vi "STP Protocol_Post_VI_Init.vi"(0 "object in":refnum<class "STP Protocol.lvclass">, 5 "Init Data":T1={"TxID"=0, "RxID"=0, "CMD"=0, "RQ Data"=[], "+veResponseCode"=160, "ResponseTimeout (S)"=0.1} {"ResponseTimeout (S)" format="%#_13g"; "+veResponseCode" format="%x"; "CMD" items=["TSW_VERSION(130)"=130, "WAIT_EVENT(132)"=132, "SEQUENCER(133)"=133, "TSW_RESET(150)"=150, "CONFIG_ECU(151)"=151, "TEST_CORE (152)"=152, "TEST_WATCHDOG (153)"=153, "TEST_MONITORING (154)"=154, "READ_MEMORY (162)"=162, "WRITE_ERASE_MEMORY (164)"=164, "COMM_EXTERNAL (190)"=190, "COMM_INTERNAL (195)"=195, "GET_ANALOG_INPUT (210)"=210, "GET_DIGITAL_INPUT (211)"=211, "GET_FREQUENCY_INPUT (212)"=212, "TEST_INPUT_STRUCTURE (214)"=214, "GENERATE_OUTPUT_SIGNAL (220)"=220, "GENERATE_SYNCHRONIZED_OUTPUT_SIGNALS (221)"=221, "eDCU_Specific (250)"=250]; "RxID" format="%.0x"; "TxID" format="%.0x"}, 7 "Socket No":u16, 11 "error in (no error)":errorcluster) -> (4 "object out":refnum<class "STP Protocol.lvclass">, 15 "error out":errorcluster)   [LabVIEW 2023, in "HardwareAbstractionLayer_LVOOP.lvlib" / "CAN Application Protocols Lib.lvlib" / "STP Protocol.lvclass"]
uses:
  STP Protocol.lvclass
  Ctrls/STP Input Data.ctl
  Ctrls/STP CMD.ctl
  Teststand Steptypes/CAN/CAN Engine/Control/CAN FGV State.ctl
  <vilib>/xnet/xnet.llb/XNET Frame CAN.ctl
  <vilib>/xnet/xnet.llb/XNET Frame Type CAN.ctl
  STP Protocol.lvclass/STP Protocol.ctl
  Teststand Steptypes/LTT_TeststandSteptypes.lvlib
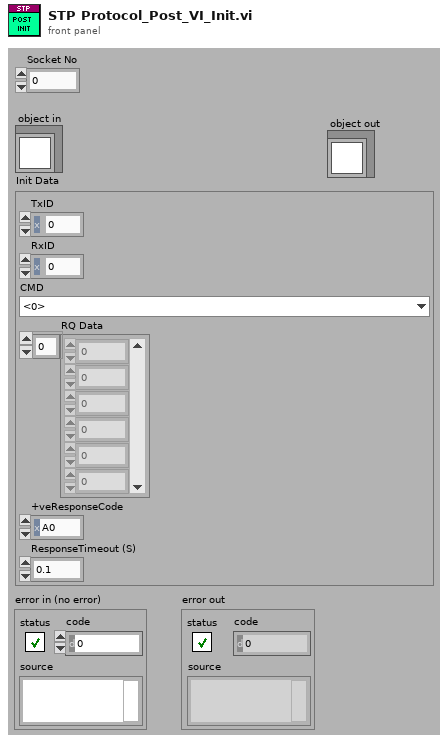
[diagram p1: front panel]
types:
  T1 = typedef "HardwareAbstractionLayer_LVOOP.lvlib/CAN Application Protocols Lib.lvlib/STP Protocol.lvclass/STP Input Data.ctl" = cluster{"TxID":u32, "RxID":u32, "CMD":T2, "RQ Data":u8[], "+veResponseCode":u8, "ResponseTimeout (S)":dbl}
  T2 = typedef "HardwareAbstractionLayer_LVOOP.lvlib/CAN Application Protocols Lib.lvlib/STP Protocol.lvclass/STP CMD.ctl" = u8
  T3 = typedef "LTT_TeststandSteptypes.lvlib/CAN FGV State.ctl" = enum16{"Init", "Get", "Set"}
  T4 = typedef "XNET Frame CAN.ctl" = cluster{"timestamp":timestamp, "payload":u8[], "identifier":u32, "type":T5, "extended?":bool, "echo?":bool}
  T5 = typedef "XNET Frame Type CAN.ctl" = u8
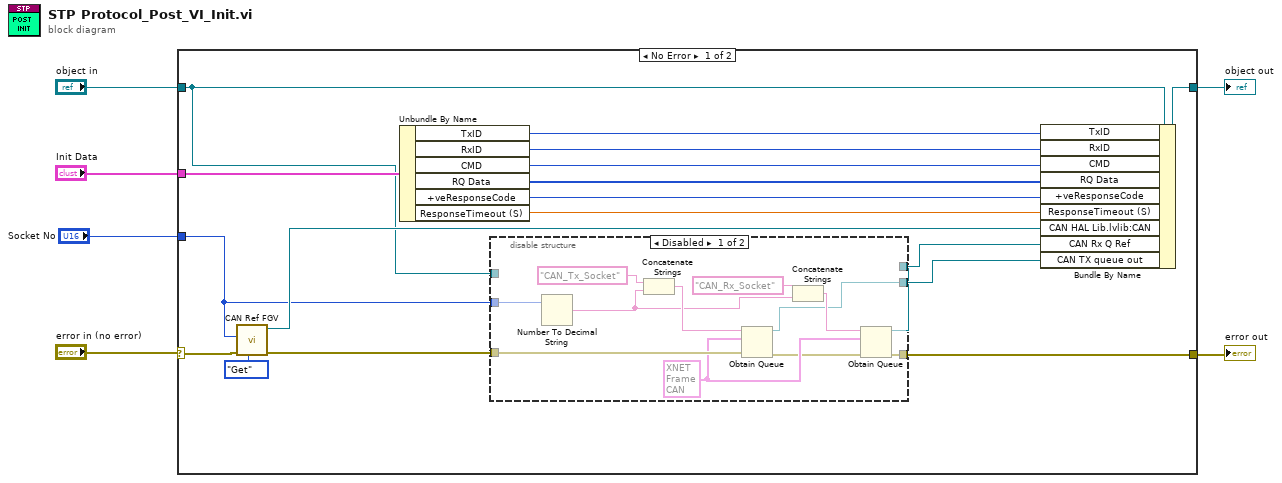
[diagram p0: block diagram]
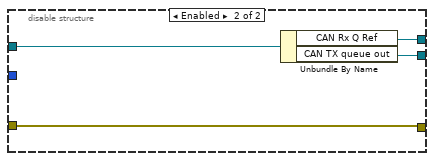
[diagram p2: hidden frame]
diagram:
  n1 = case shown="No Error" "error in (no error)" {
    selector: "error in (no error)" -> [w15 w40]
    tunnel: "object in" -> [w7 w41]
    tunnel: [w23 w41] -> w5
    tunnel: [w10 w40] -> w3
    tunnel: "Init Data" -> [w18 _]
    tunnel: "Socket No" -> [w11 _]
    frame No Error {
      n2 = call "CAN Ref FGV.vi"("CAN FGV State"=CAN_FGV_State."Get", "error in"=w15, "Socket No"=w11) -> ("error out"=w12:errorcluster, "object out"=w13:refnum<class "NI-XNET.lvclass">)  [unwired: 6 in, 1 out]
      n3 = Unbundle By Name(w18) -> ("TxID"=w22:u32, "RxID"=w21:u32, "CMD"=w20:T2, "RQ Data"=w19:u8[], "+veResponseCode"=w17:u8, "ResponseTimeout (S)"=w16:dbl)
      n4 = disable-structure shown="Disabled" {
        disable-tunnel: w12 -> [w35 w36]
        disable-tunnel: w11 -> [w34 _]
        disable-tunnel: [w28 w36] -> w10
        disable-tunnel: [w25 w37] -> w9
        disable-tunnel: [w24 w38] -> w8
        disable-tunnel: w7 -> [_ w39]
        frame Disabled {
          w29 = T4 {"timestamp"=timestamp(0 s since 1904-01-01), "payload"=[], "identifier"=0, "type"=0, "extended?"=FALSE, "echo?"=FALSE} ("CAN frame")
          n5 = Number To Decimal String(number=w34) -> (decimal integer string=w26:string)  [unwired: 1 in]
          n6 = Concatenate Strings("CAN_Tx_Socket" ("name (unnamed)"), w26) -> (w33:string)
          n7 = Obtain Queue(name (unnamed)=w33, element data type=w29, error in (no error)=w35) -> (queue out=w25:refnum<queue>, error out=w27:errorcluster)  [unwired: 2 in, 1 out]
          n8 = Concatenate Strings("CAN_Rx_Socket" ("name (unnamed)"), w26) -> (w31:string)
          n9 = Obtain Queue(name (unnamed)=w31, element data type=w29, error in (no error)=w27) -> (queue out=w24:refnum<queue>, error out=w28:errorcluster)  [unwired: 2 in, 1 out]
        }
        frame Enabled {
          n10 = Unbundle By Name(w39) -> ("CAN Rx Q Ref"=w38:refnum<queue>, "CAN TX queue out"=w37:refnum<queue>)
        }
      }
      n11 = Bundle By Name(cluster=w7, "TxID"=w22, "RxID"=w21, "CMD"=w20, "RQ Data"=w19, "+veResponseCode"=w17, "ResponseTimeout (S)"=w16, "CAN HAL Lib.lvlib:CAN"=w13, "CAN Rx Q Ref"=w8, "CAN TX queue out"=w9) -> (w23:refnum<class "STP Protocol.lvclass">)
    }
    frame Error {
    }
  }
  "object out" <- w5
  "error out" <- w3
